vi "TempPath.vi"(2 "change":bool, 3 "stripped path":path) -> (0 "stripped path 2":path)   [LabVIEW 2009]
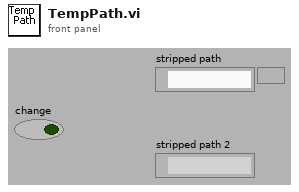
[diagram p1: front panel]
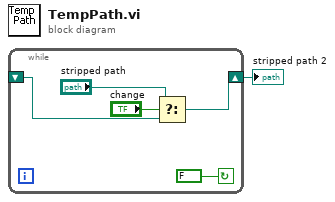
[diagram p0: block diagram]
diagram:
  n1 = while {
    shift-right: [w6] -> w1
    shift-left: _ -> [w2]
    stop <- FALSE continue-if-true
    n2 = Select(t="stripped path", s="change", f=w2) -> (s? t:f=w6:path)
  }
  "stripped path 2" <- w1
